vi "Write Stop Viewer UE.vi"(8 "error in (no error)":errorcluster, 10 "Stop Viewer UE":refnum<user-event>, 11 "ResultsViewer in":refnum<class "ResultsViewer.lvclass">) -> (0 "error out":errorcluster, 3 "ResultsViewer out":refnum<class "ResultsViewer.lvclass">)   [LabVIEW 2019, in "ResultsViewer.lvlib" / "ResultsViewer.lvclass"]
uses:
  ResultsViewer.lvclass
  <vilib>/ActorFramework/Message Enqueuer/Message Enqueuer.lvclass
  ResultsViewer.lvclass/ResultsViewer.ctl
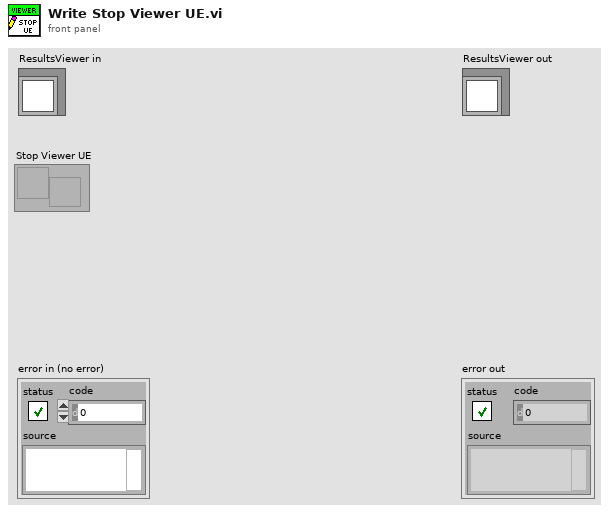
[diagram p1: front panel]
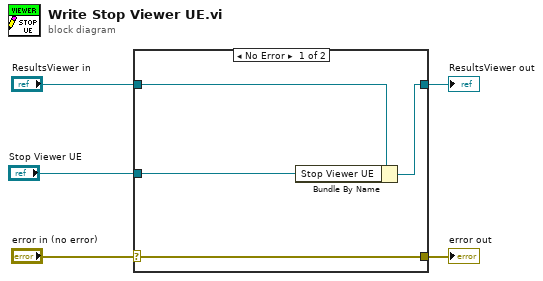
[diagram p0: block diagram]
diagram:
  n1 = case shown="No Error" "error in (no error)" {
    selector: "error in (no error)" -> [w9 w10]
    tunnel: [w9 w10] -> w4
    tunnel: [w7 w11] -> w2
    tunnel: "ResultsViewer in" -> [w8 w11]
    tunnel: "Stop Viewer UE" -> [w6 _]
    frame No Error {
      n2 = Bundle By Name(cluster=w8, "Stop Viewer UE"=w6) -> (w7:refnum<class "ResultsViewer.lvclass">)
    }
    frame Error {
    }
  }
  "error out" <- w4
  "ResultsViewer out" <- w2
